vi "GetDLLPaths.vi"() -> (1 "PCO_Conv_Path":path, 2 "PCO_Recorder_Path":path, 3 "SC2_Cam_Path":path)   [LabVIEW 2020]
doc: "Returns the absolut paths of the pco DLLs according to the LabVIEW Bitness\nSC2_Cam.dll\nPCO_Recorder.dll\nPCO_Conv.dll"
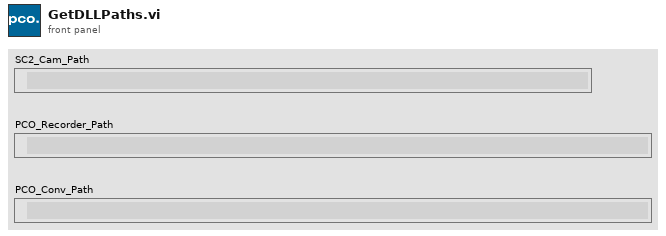
[diagram p1: front panel]
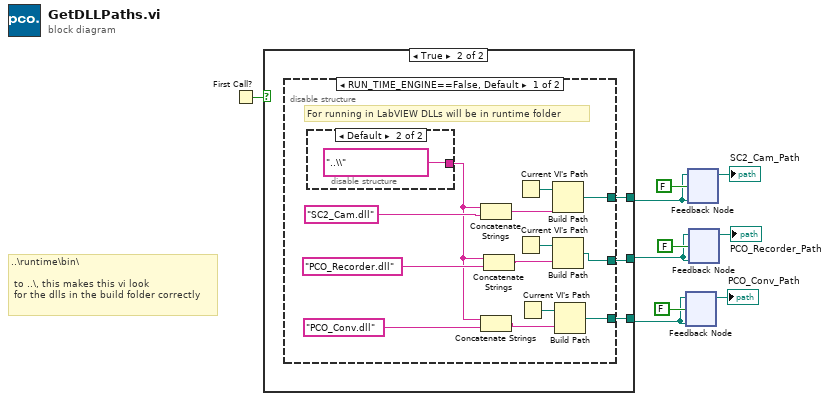
[diagram p0: block diagram]
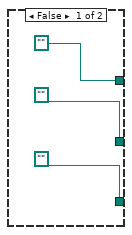
[diagram p2: hidden frame]
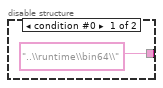
[diagram p3: hidden frame]
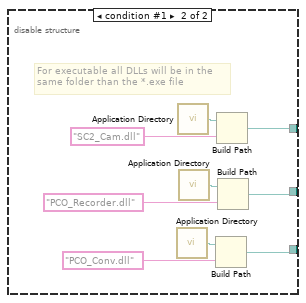
[diagram p4: hidden frame]
diagram:
  # "..\\runtime\\bin\\\n\n to ..\\, this makes this vi look\n for the dlls in the build folder correctly"
  n1 = First Call?() -> (First Call?: T/F=w7:bool)
  n2 = case shown="True" w7 {
    tunnel: [path "" w16] -> w8
    tunnel: [path "" w15] -> w1
    tunnel: [path "" w14] -> w2
    frame False {
    }
    frame True {
      n3 = disable-structure shown="RUN_TIME_ENGINE==False, Default" {
        disable-tunnel: [w19 w38] -> w16
        disable-tunnel: [w18 w35] -> w15
        disable-tunnel: [w17 w34] -> w14
        frame condition #0 (active) {
          # "For running in LabVIEW DLLs will be in runtime folder"
          n4 = disable-structure shown="Default" {
            disable-tunnel: ["..\\runtime\\bin64\\" "..\\"] -> w24
            frame condition #0 {
            }
            frame condition #1 (active) {
            }
          }
          n5 = Concatenate Strings(w24, "SC2_Cam.dll") -> (w27:string)
          n6 = Concatenate Strings(w24, "PCO_Conv.dll") -> (w21:string)
          n7 = Concatenate Strings(w24, "PCO_Recorder.dll") -> (w20:string)
          n8 = Current VI's Path() -> (path=w29:path)
          n9 = Current VI's Path() -> (path=w23:path)
          n10 = Current VI's Path() -> (path=w22:path)
          n11 = Build Path(base path=w29, name or relative path=w27) -> (appended path=w19:path)
          n12 = Build Path(base path=w23, name or relative path=w20) -> (appended path=w18:path)
          n13 = Build Path(base path=w22, name or relative path=w21) -> (appended path=w17:path)
        }
        frame condition #1 {
          # "For executable all DLLs will be in the \nsame folder than the *.exe file"
          n14 = call "Application Directory.vi"() -> ("Application Directory"=w36:path)
          n15 = call "Application Directory.vi"() -> ("Application Directory"=w40:path)
          n16 = call "Application Directory.vi"() -> ("Application Directory"=w37:path)
          n17 = Build Path(base path=w36, name or relative path="PCO_Conv.dll") -> (appended path=w34:path)
          n18 = Build Path(base path=w40, name or relative path="SC2_Cam.dll") -> (appended path=w38:path)
          n19 = Build Path(base path=w37, name or relative path="PCO_Recorder.dll") -> (appended path=w35:path)
        }
      }
    }
  }
  n20 = feedback #1(w2) -> (→"PCO_Conv_Path":path)
  n21 = feedback-in #1(w2, FALSE) -> ()
  n22 = feedback #2(w8) -> (→"SC2_Cam_Path":path)
  n23 = feedback-in #2(w8, FALSE) -> ()
  n24 = feedback #3(w1) -> (→"PCO_Recorder_Path":path)
  n25 = feedback-in #3(w1, FALSE) -> ()
